vi "LogStringToSDCard.vi"(8 "Log string":string, 9 "SerialPortRef":T1) -> (3 "SerialPortRef out":T1)   [LabVIEW 2014]
uses:
  <vilib>/Rock Robotics/WPI/SerialPort/WPI_SerialPortRef.ctl
panel:
  out "error out":errorcluster
  in  "error in (no error)":errorcluster
  # "Cannot contain line breaks or the character 0x00"
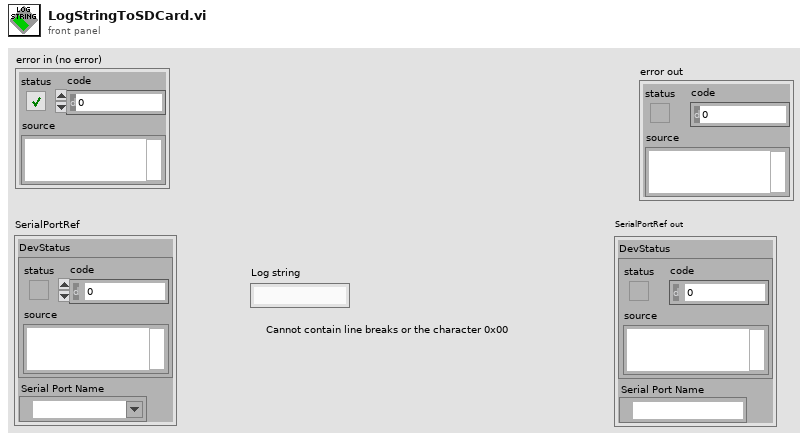
[diagram p1: front panel]
types:
  T1 = typedef "WPI_SerialPortRef.ctl" = cluster{"DevStatus":errorcluster, "Serial Port Name":refnum<visa-resource-name>}
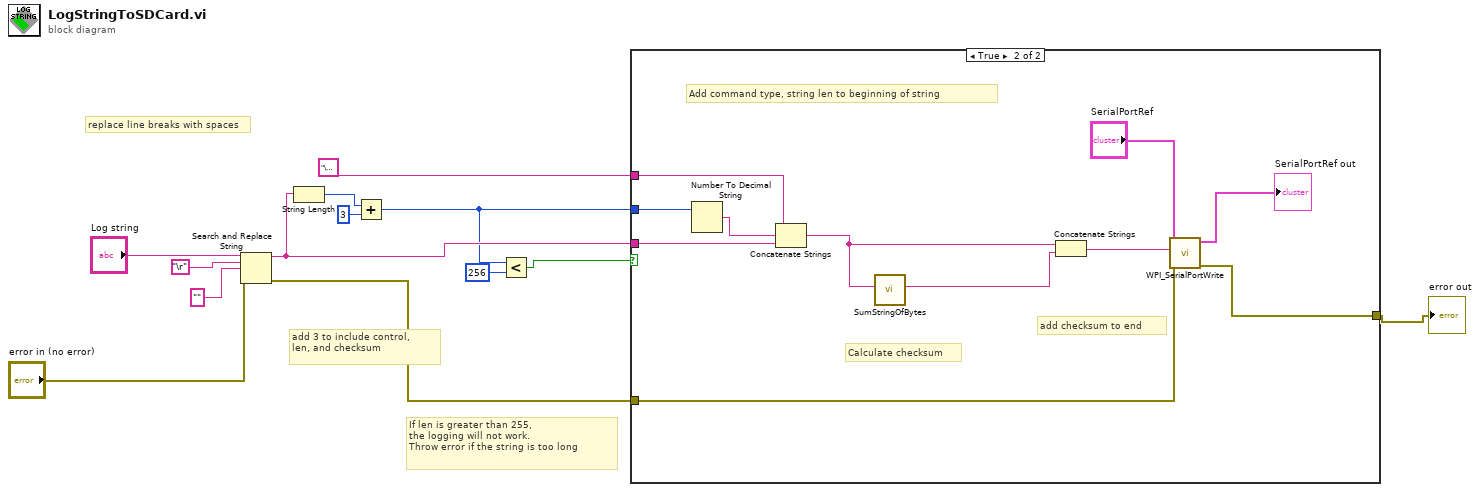
[diagram p0: block diagram]
diagram:
  # "If len is greater than 255,\nthe logging will not work.\nThrow error if the string is too long"
  # "add 3 to include control, \nlen, and checksum"
  # "replace line breaks with spaces"
  n1 = Search and Replace String(input string="Log string", search string="\r", replace string="" ("replace string (\"\")"), error in="error in (no error)") -> (result string=w5:string, error out=w9:errorcluster)  [unwired: 4 in, 2 out]
  n2 = String Length(string=w5) -> (length=w7:i32)
  n3 = Add(x=w7, y=3) -> (x+y=w3:i32)
  n4 = Less?(x=w3, y=256) -> (x < y?=w1:bool)
  n5 = case shown="True" w1 {
    tunnel: w9 -> [_ w22]
    tunnel: "\u0001" ("string") -> [_ w21]
    tunnel: w3 -> [_ w20]
    tunnel: w5 -> [_ w15]
    tunnel: [_ w14] -> w4
    frame False {
    }
    frame True {
      # "add checksum to end"
      # "Add command type, string len to beginning of string"
      # "Calculate checksum"
      n6 = Number To Decimal String(number=w20) -> (decimal integer string=w19:string)  [unwired: 1 in]
      n7 = Concatenate Strings(w21, w19, w15) -> (w18:string)
      n8 = call "SumStringOfBytes.vi"("String Of Bytes"=w18) -> ("SumAsString"=w17:string)  [unwired: 10 in]
      n9 = Concatenate Strings(w18, w17) -> (w16:string)
      n10 = call <vilib>:"WPI_SerialPortWrite.vi"("error in (no error)"=w22, "Buffer"=w16, "SerialPortRef"="SerialPortRef") -> ("error out"=w14:errorcluster, "SerialPortRef"=→"SerialPortRef out":T1)  [unwired: 6 in, 1 out]
    }
  }
  "error out" <- w4
